vi "presure PA.vi"(11 "Volte":dbl) -> (0 "presure String":string, 1 "Presure dbl":dbl, 3 "err presure":bool, 4 "presure String 2":string)   [LabVIEW 2016, in "Library.lvlib"]
uses:
  Granule-2000AT/PC/Library.lvlib
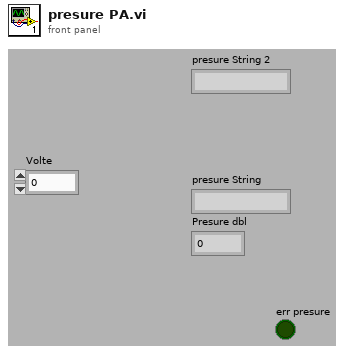
[diagram p1: front panel]
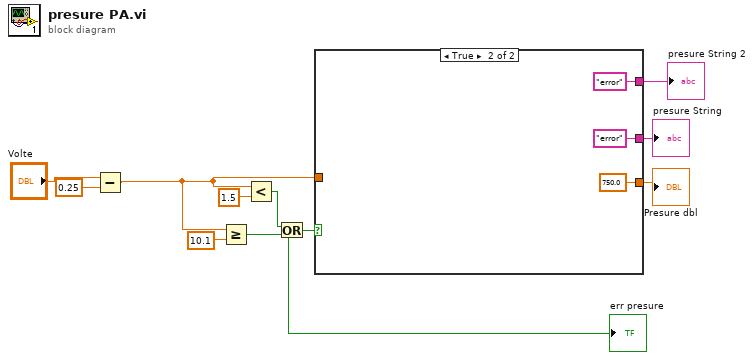
[diagram p0: block diagram]
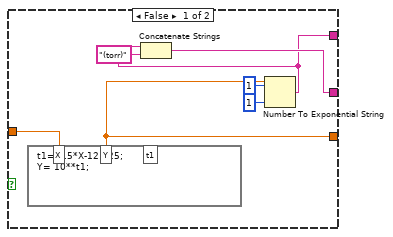
[diagram p2: hidden frame]
diagram:
  n1 = Subtract(x="Volte", y=0.25) -> (x-y=w3:dbl)
  n2 = Greater Or Equal?(x=w3, y=10.1) -> (x >= y?=w9:bool)
  n3 = Less?(x=w3, y=1.5) -> (x < y?=w8:bool)
  n4 = Or(x=w8, y=w9) -> (x .or. y?=w7:bool)
  "err presure" <- w7
  n5 = case shown="True" w7 {
    tunnel: w3 -> [w18 _]
    tunnel: [w13 "error"] -> w6
    tunnel: [w15 750.0 ("Y")] -> w5
    tunnel: [w12 "error"] -> w4
    frame False {
      n6 = formula code="t1= 1.5*X-12.125;\nY= 10**t1;"("X"=w18) -> ("Y"=w15:dbl)  [unwired: 1 out]
      n7 = Number To Exponential String(number=w15, precision (6)=i16 1, 3:i16 1 ("width (-)")) -> (E-format string=w12:string)  [unwired: 1 in]
      n8 = Concatenate Strings(w12, "(torr)" ("string")) -> (w13:string)
    }
    frame True {
    }
  }
  "presure String" <- w6
  "Presure dbl" <- w5
  "presure String 2" <- w4
